vi "Weibull Random.vi"(6 "seed":i32=-1, 7 "reset":bool, 9 "b":dbl=3.0, 10 "a":dbl=1.0, 11 "samples":i32=128) -> (0 "error":i32, 3 "Weibull random numbers":dbl[](array[numeric]))   [LabVIEW 2017, in "NI_Gmath.lvlib"]
doc: "Generates random values from a variate X, where X describes the selected distribution type. You must manually select the polymorphic instance to use."
uses:
  NI_Gmath.lvlib
  st_error_code.ctl
panel:
  # "Weibull Random"
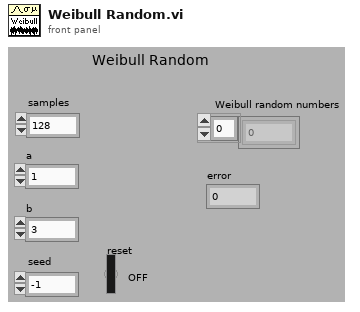
[diagram p1: front panel]
types:
  T1 = typedef "NI_Gmath.lvlib/st_error_code.ctl" = i32
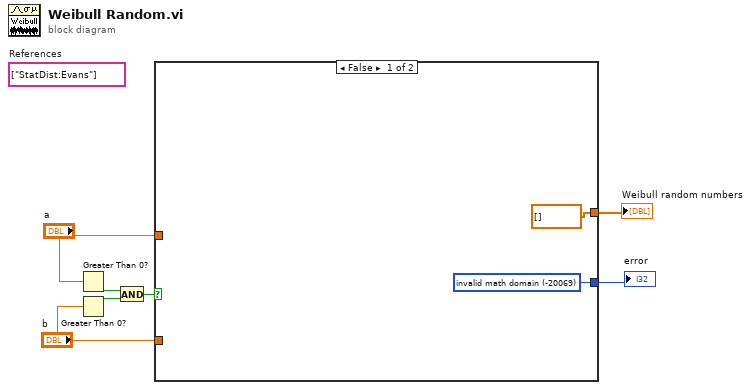
[diagram p0: block diagram]
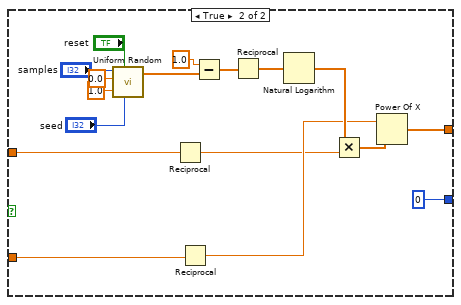
[diagram p2: hidden frame]
diagram:
  (unwired) string[] ["StatDist:Evans"]  # References
  n1 = Greater Than 0?(x="a") -> (x > 0?=w7:bool)
  n2 = Greater Than 0?(x="b") -> (x > 0?=w5:bool)
  n3 = And(x=w7, y=w5) -> (x .and. y?=w6:bool)
  n4 = case shown="False" w6 {
    tunnel: "b" -> [_ w25]
    tunnel: [w9 0 ("invalid math domain")] -> w1
    tunnel: [dbl[] [] w10] -> w2
    tunnel: "a" -> [_ w12]
    frame False {
      w9 = T1 -20069 items=["invalid math domain"=-20069, "Fourier interpolation size m >= n"=-20070, "empty array"=-20003] ("stat interp error code")
    }
    frame True {
      n5 = call "Uniform Random.vi"("seed"="seed", "reset"="reset", "xmax"=1.0, "xmin"=0.0, "samples"="samples") -> ("uniform random data"=w14:dbl[])  [unwired: 5 in, 1 out]
      n6 = Reciprocal(x=w12) -> (1/x=w11:dbl)
      n7 = Reciprocal(x=w25) -> (1/x=w13:dbl)
      n8 = Subtract(x=1.0, y=w14) -> (x-y=w18:dbl[])
      n9 = Reciprocal(x=w18) -> (1/x=w17:dbl[])
      n10 = Natural Logarithm(1:w17) -> (0:w16:dbl[])
      n11 = Multiply(x=w16, y=w11) -> (x*y=w15:dbl[])
      n12 = Power Of X(1:w15, 2:w13) -> (0:w10:dbl[])
    }
  }
  "error" <- w1
  "Weibull random numbers" <- w2
